vi "create_shared_link-basic.vi"(8 "error in (no error)":errorcluster, 10 "short_url":bool, 11 "path":string) -> (0 "error out":errorcluster, 3 "url":string)   [LabVIEW 2015, in "lv-dropbox.lvlib" / "v2.lvlib"]
uses:
  v2.lvlib
  <vilib>/httpClient/POSTBuffer.vi
  <vilib>/httpClient/LabVIEWHTTPClient.lvlib
  lv-dropbox.lvlib
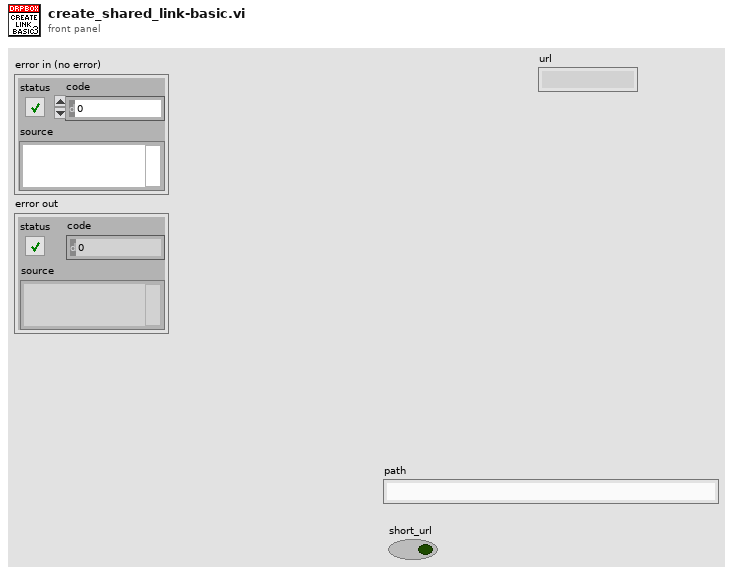
[diagram p1: front panel]
types:
  T1 = cluster{"url":string, "visibility":cluster{".tag":string}, "path":string}
  T2 = typedef "LabVIEWHTTPClient.lvlib/ClientHandle.ctl" = refnum<k1>
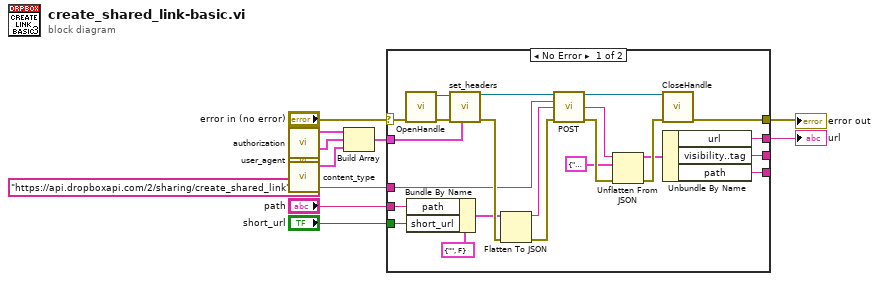
[diagram p0: block diagram]
diagram:
  n1 = call "authorization.vi"() -> ("header"=w7:cluster{"header":string, "value":string})  [unwired: 11 in]
  n2 = call "user_agent.vi"() -> ("header"=w6:cluster{"header":string, "value":string})  [unwired: 11 in]
  n3 = call "content_type.vi"() -> ("header"=w8:cluster{"header":string, "value":string})  [unwired: 11 in]
  n4 = Build Array(w7, w6, w8) -> (w9:cluster{"header":string, "value":string}[])
  n5 = case shown="No Error" "error in (no error)" {
    selector: "error in (no error)" -> [w27 w34]
    tunnel: "https://api.dropboxapi.com/2/sharing/create_shared_link" ("url") -> [w29 _]
    tunnel: w9 -> [w25 _]
    tunnel: [w21 w34] -> w5
    tunnel: "path" -> [w17 _]
    tunnel: "short_url" -> [w16 _]
    tunnel: [w13 _] -> w1
    tunnel: [w12 _] -> _
    tunnel: [w11 _] -> _
    frame No Error {
      n6 = call <vilib>:"OpenHandle.vi"("error in (no error)"=w27) -> ("client handle out"=w28:T2, "error out"=w26:errorcluster)  [unwired: 13 in]
      n7 = Bundle By Name(cluster=cluster{"path":string, "short_url":bool} {"path"="", "short_url"=FALSE}, "path"=w17, "short_url"=w16) -> (w18:cluster{"path":string, "short_url":bool})
      n8 = call "set_headers.vi"("header_value []"=w25, "error in (no error)"=w26, "client_handle in"=w28) -> ("error out"=w33:errorcluster, "client_handle out"=w24:T2)  [unwired: 7 in]
      n9 = Flatten To JSON(anything=w18, error in (no error)=w33) -> (JSON string=w15:string, 11:w32:errorcluster)  [unwired: 1 in]
      n10 = call-poly <vilib>:"POST.vi"("client handle"=w24, "url"=w29, "buffer"=w15, "error in (no error)"=w32) -> ("client handle out"=w23:T2, "body"=w22:string, "error out"=w31:errorcluster)  [unwired: 8 in, 1 out]
      n11 = Unflatten From JSON(JSON string=w22, type and defaults=T1 {"url"="", "visibility"={".tag"=""}, "path"=""}, error in (no error)=w31) -> (value=w14:T1, error out=w30:errorcluster)  [unwired: 4 in]
      n12 = call <vilib>:"CloseHandle.vi"("client handle"=w23, "error in (no error)"=w30) -> ("error out"=w21:errorcluster)  [unwired: 13 in]
      n13 = Unbundle By Name(w14) -> ("url"=w13:string, "visibility..tag"=w12:string, "path"=w11:string)
    }
    frame Error {
    }
  }
  "error out" <- w5
  "url" <- w1
